vi "Destroy.vi"(0 "reference in":refnum<class "Power Supply.lvclass">, 5 "error in (no error)":errorcluster) -> (14 "reference out":refnum<class "Power Supply.lvclass">, 19 "error out":errorcluster)   [LabVIEW 2017, in "Power Supply.lvclass"]
uses:
  Power Supply.lvclass
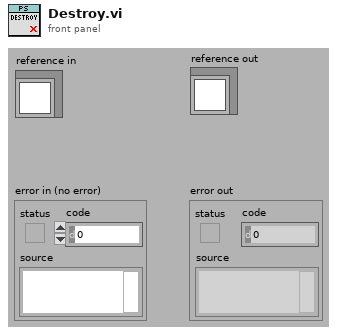
[diagram p1: front panel]
types:
  T1 = typedef "Power Supply.lvclass/ObjectAttributes.ctl" = cluster{"Power Supply Chain VISA Session":refnum<visa-resource-name>, "Power Supply Chain Address":i16, "Power Supply Open/Close Status":bool, "Power Supply Voltage Setting":dbl, "Power Supply Current Setting":dbl, "Power Supply Voltage Reading":dbl, "Power Supply Current Reading":dbl, "Power Supply Status":T2, "Power Supply Error":T3, "Fault Register":u8, "Power Supply Error":bool}
  T2 = typedef "Power Supply.lvclass/Power Supply Status.ctl" = enum16{"Closed", "Open"}
  T3 = typedef "Power Supply.lvclass/Power Supply Error.ctl" = enum16{"None", "Read Error"}
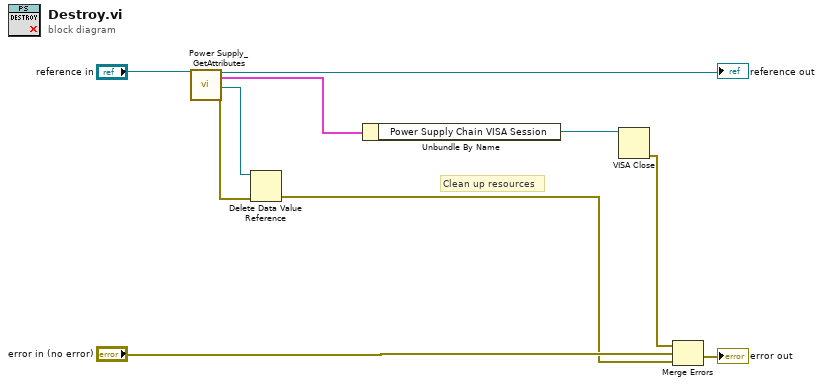
[diagram p0: block diagram]
diagram:
  # "Clean up resources"
  n1 = call "Power Supply_GetAttributes.vi"("reference in"="reference in") -> ("reference out"=→"reference out":refnum<class "Power Supply.lvclass">, "Data"=w4:T1, "DataRef"=w6:refnum<data-value>, "error out"=w7:errorcluster)  [unwired: 15 in]
  n2 = Delete Data Value Reference(data value reference=w6, error in=w7) -> (error out=w2:errorcluster)  [unwired: 1 out]
  n3 = Unbundle By Name(w4) -> ("Power Supply Chain VISA Session"=w3:refnum<visa-resource-name>)
  n4 = VISA Close(VISA resource name=w3) -> (error out=w1:errorcluster)  [unwired: 1 in]
  n5 = Merge Errors(w1, "error in (no error)", w2) -> (→"error out":errorcluster)
